vi "DualEncoder.vi"(8 "error in (no error)":errorcluster, 11 "Reset?":bool) -> (0 "error out":errorcluster, 1 "Distance Right (in)":dbl, 2 "Distance Left (in)":dbl, 3 "Total Distance (in)":dbl)   [LabVIEW 2012]
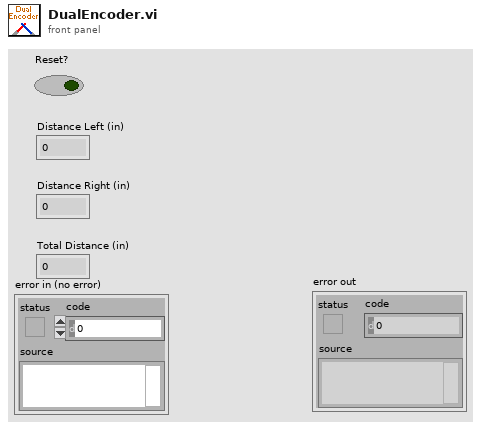
[diagram p1: front panel]
types:
  T1 = typedef "WPI_EncoderDevRef.ctl" = cluster{"DevStatus":errorcluster, "EncoderIndex":T2, "CounterIndex":T3, "DistancePerCount":dbl, "Decoding Type":T4}
  T2 = typedef "FPGA_EncoderIdx.ctl" = enum8{"Enc 0", "Enc 1", "Enc 2", "Enc 3", "Invalid"}
  T3 = typedef "FPGA_CounterCtrSystemIndex.ctl" = enum8{"Ctr 0", "Ctr 1", "Ctr 2", "Ctr 3", "Ctr 4", "Ctr 5", "Ctr 6", "Ctr 7", "Invalid"}
  T4 = typedef "WPI_EncoderType.ctl" = enum16{"1x", "2x", "4x"}
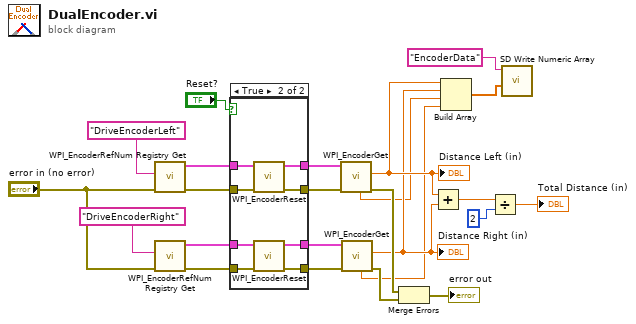
[diagram p0: block diagram]
diagram:
  n1 = call <vilib>:"WPI_EncoderRefNum Registry Get.vi"("error in (no error)"="error in (no error)", "refnum name"="DriveEncoderLeft") -> ("error out"=w18:errorcluster, "EncoderDevRef"=w19:T1)  [unwired: 8 in]
  n2 = call <vilib>:"WPI_EncoderRefNum Registry Get.vi"("error in (no error)"="error in (no error)", "refnum name"="DriveEncoderRight") -> ("error out"=w20:errorcluster, "EncoderDevRef"=w21:T1)  [unwired: 8 in]
  n3 = case shown="True" "Reset?" {
    tunnel: w21 -> [w26 w36]
    tunnel: w20 -> [w25 w35]
    tunnel: w19 -> [w28 w34]
    tunnel: w18 -> [w27 w33]
    tunnel: [w28 w32] -> w16
    tunnel: [w27 w31] -> w15
    tunnel: [w26 w30] -> w14
    tunnel: [w25 w29] -> w13
    frame False {
    }
    frame True {
      n4 = call <vilib>:"WPI_EncoderReset.vi"("error in (no error)"=w33, "EncoderDevRef"=w34) -> ("error out"=w31:errorcluster, "EncoderDevRef"=w32:T1)  [unwired: 8 in]
      n5 = call <vilib>:"WPI_EncoderReset.vi"("error in (no error)"=w35, "EncoderDevRef"=w36) -> ("error out"=w29:errorcluster, "EncoderDevRef"=w30:T1)  [unwired: 8 in]
    }
  }
  n6 = call <vilib>:"WPI_EncoderGet.vi"("error in (no error)"=w15, "EncoderDevRef"=w16) -> ("error out"=w9:errorcluster, "Distance"=w4:dbl, "Rate"=w2:dbl)  [unwired: 4 in, 3 out]
  "Distance Left (in)" <- w4
  n7 = call <vilib>:"WPI_EncoderGet.vi"("error in (no error)"=w13, "EncoderDevRef"=w14) -> ("error out"=w8:errorcluster, "Distance"=w3:dbl, "Rate"=w1:dbl)  [unwired: 4 in, 3 out]
  "Distance Right (in)" <- w3
  n8 = Merge Errors(w9, w8) -> (→"error out":errorcluster)
  n9 = Add(x=w4, y=w3) -> (x+y=w11:dbl)
  n10 = Build Array(w4, w3, w2, w1) -> (w5:dbl[])
  n11 = Divide(x=w11, y=2) -> (x/y=→"Total Distance (in)":dbl)
  n12 = call <vilib>:"SD Write Numeric Array.vi"("Numeric Array"=w5, "Name"="EncoderData") -> ()  [unwired: 8 in, 2 out]
